vi "User Access Level FGV Unit Test.vi"() -> ()   [LabVIEW 2024]
uses:
  User Level Cmd.ctl
panel:
  in  "Access Secure Area":bool
  out "Error Out":errorcluster
  in  "Error In":errorcluster
  in  "Current User":string
  in  "Set User Access Level":bool
  in  "stop":bool
  # "1.  Set access level for current user."
  # "2.  Test access level by verifying the appropriate dialog message."
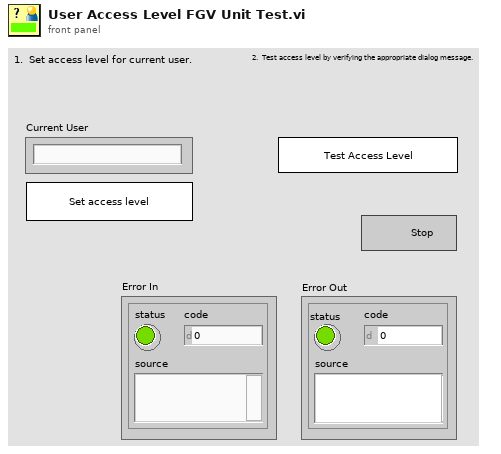
[diagram p1: front panel]
types:
  T1 = typedef "User Level Cmd.ctl" = enum16{"Read User Access Level File", "Set Current Access Level", "Get Current Access Level"}
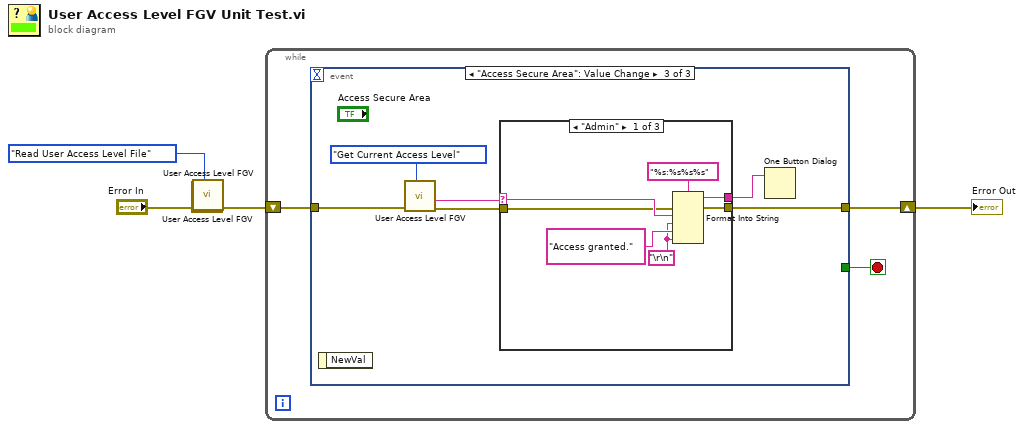
[diagram p0: block diagram]
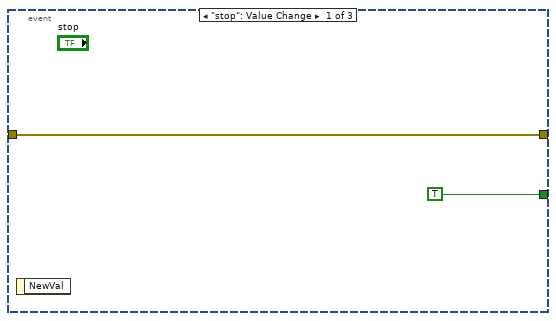
[diagram p2: hidden frame]
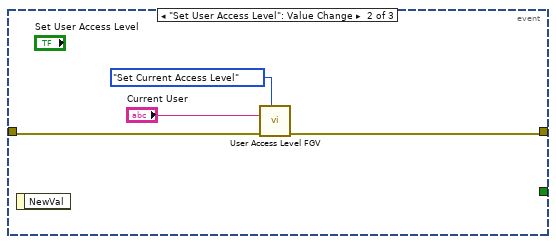
[diagram p3: hidden frame]
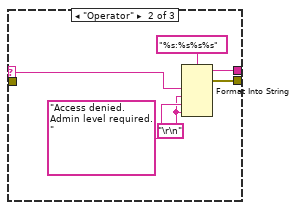
[diagram p4: hidden frame]
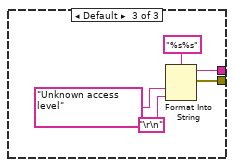
[diagram p5: hidden frame]
diagram:
  n1 = call "User Access Level FGV.vi"() -> ()  [unwired: 10 in, 2 out]
  n2 = call "User Access Level FGV.vi"("User Level Control"=User_Level_Cmd."Read User Access Level File", "Error In"="Error In") -> ("Error Out"=w2:errorcluster)  [unwired: 8 in, 1 out]
  n3 = while {
    shift-right: [w5] -> w4
    shift-left: w2 -> [w6]
    stop <- w7 stop-if-true
    n4 = event shown="[2] \"Access Secure Area\": Value Change" {
      selector: _ -> [_ _ _]
      dyn-events: _ -> [_ _ _]
      timeout: _ -> [_ _ _]
      tunnel: [TRUE ("stop") _ _] -> w7
      tunnel: w6 -> [w8 w12 w17]
      tunnel: [w8 w11 w19] -> w5
      event "stop": Value Change {
        n5 = event-data() -> ()  [unwired: 1 in, 1 out]
      }
      event "Set User Access Level": Value Change {
        n6 = event-data() -> ()  [unwired: 1 in, 1 out]
        n7 = call "User Access Level FGV.vi"("User Level Control"=User_Level_Cmd."Set Current Access Level", "Error In"=w12, "User Name"="Current User") -> ("Error Out"=w11:errorcluster)  [unwired: 7 in, 1 out]
      }
      event "Access Secure Area": Value Change {
        n8 = event-data() -> ()  [unwired: 1 in, 1 out]
        n9 = call "User Access Level FGV.vi"("User Level Control"=User_Level_Cmd."Get Current Access Level", "Error In"=w17) -> ("Error Out"=w16:errorcluster, "User Level"=w15:string)  [unwired: 8 in]
        n10 = case shown="\"Admin\"" w15 {
          selector: w15 -> [w26 w32 _]
          tunnel: [w25 w31 w37] -> w19
          tunnel: [w21 w27 w35] -> w18
          tunnel: w16 -> [w20 _ _]
          frame "Admin" {
            w23 = "\r\n"
            n11 = Format Into String(format string="%s:%s%s%s", error in=w20, w26, w23, "Access granted." ("message"), w23) -> (resulting string=w21:string, error out=w25:errorcluster)  [unwired: 1 in]
          }
          frame "Operator" {
            w29 = "\r\n"
            n12 = Format Into String(format string="%s:%s%s%s", w32, w29, "Access denied.  Admin level required." ("message"), w29) -> (resulting string=w27:string, error out=w31:errorcluster)  [unwired: 2 in]
          }
          frame Default {
            n13 = Format Into String(format string="%s%s", "Unknown access level" ("message"), "\r\n") -> (resulting string=w35:string, error out=w37:errorcluster)  [unwired: 2 in]
          }
        }
        n14 = One Button Dialog(message=w18) -> ()  [unwired: 1 in, 1 out]
      }
    }
  }
  "Error Out" <- w4
